vi "1000m_frame.vi"() -> ()   [LabVIEW 2017]
uses:
  <vilib>/gmath/NI_Gmath.lvlib
panel:
  out "normált eredõ SNR":cluster{dbl[], dbl[]}(graph)
  out "normált X SNR (+1 felharmonikus)":cluster{dbl[], dbl[]}(graph)
  out "normált X SNR":cluster{dbl[], dbl[]}(graph)
  out "r 8":dbl format="%.7g"
  out "r 7":dbl format="%.7g"
  out "r 6":dbl format="%.7g"
  out "r 5":dbl format="%.7g"
  out "r 4":dbl format="%.7g"
  out "r 3":dbl format="%.7g"
  out "r 2":dbl format="%.7g"
  out "r":dbl format="%.7g"
  out "impulse szum/mean":cluster{"X":dbl, "Y":dbl}[](graph)
  in  "felharmonikus N":i32=2
  in  "SNR window width [Hz]":dbl=0.2 format="%#_13g"
  out "impulse mean":cluster{"X":dbl, "Y":dbl}[](graph)
  out "impulse szum":cluster{"X":dbl, "Y":dbl}[](graph)
  out "impulse sd":cluster{"X":dbl, "Y":dbl}[](graph)
  out "impulse szum/time (egész jó)":cluster{"X":dbl, "Y":dbl}[](graph)
  out "X SNR (+1 felharmonikus)":cluster{"X":dbl, "Y":dbl}[](graph)
  out "resultant SNR":cluster{"X":dbl, "Y":dbl}[](graph)
  out "X SNR":cluster{"X":dbl, "Y":dbl}[](graph)
  in  "Path":path=path "C:/Users/Lenovo/Desktop/szakdoga/data/pálya/1000m"
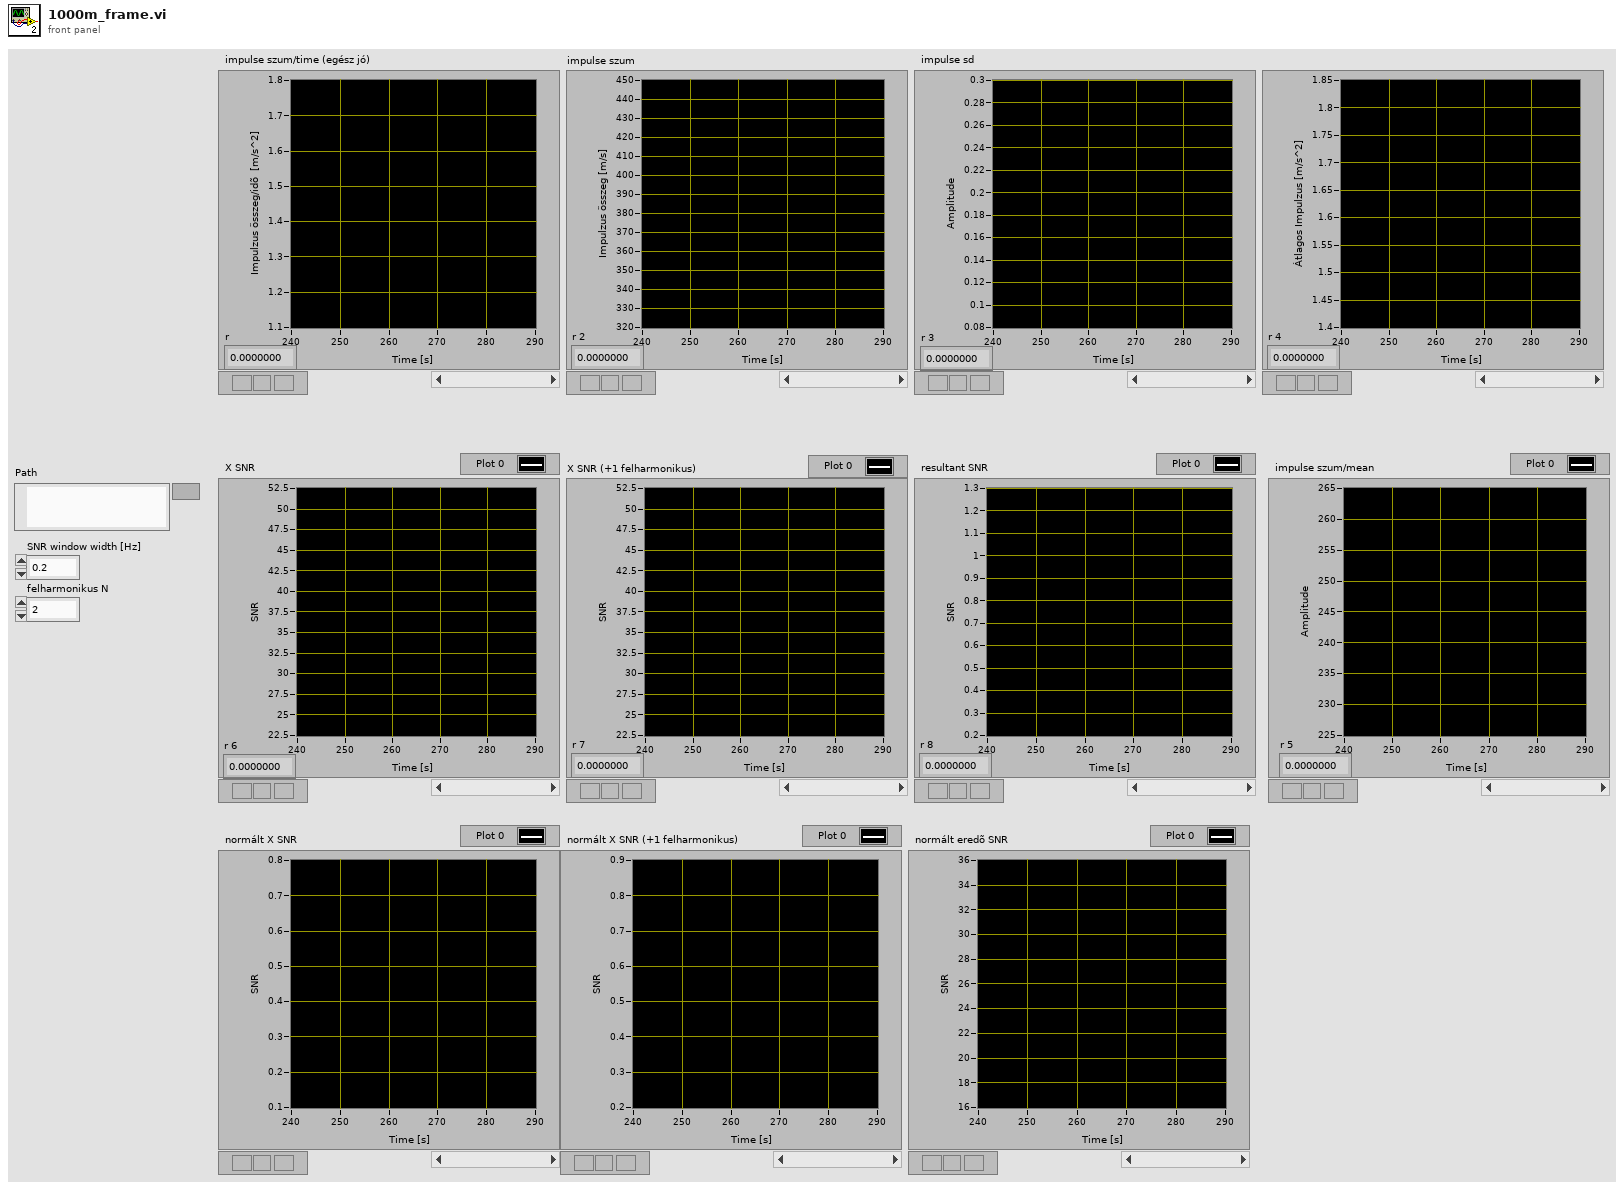
[diagram p1: front panel]
types:
  T1 = cluster{cluster{dbl, "impulse szum/time":dbl}[], cluster{dbl, "impulse  szum":dbl}[], cluster{dbl, "impulse standard deviation":dbl}[], cluster{dbl, "impulse mean":dbl}[], cluster{dbl, "X SNR 1":dbl}[], cluster{dbl, "X SNR 2":dbl}[], cluster{dbl, "X SNR 3":dbl}[], cluster{dbl, "impulse szum/avg":dbl}[]}
  T2 = cluster{cluster{dbl, dbl}[], cluster{dbl, "impulse  szum":dbl}[], cluster{dbl, "impulse standard deviation":dbl}[], cluster{dbl, "impulse mean":dbl}[], cluster{dbl, dbl}[], cluster{dbl, dbl}[], cluster{dbl, dbl}[], cluster{dbl, "impulse szum/mean":dbl}[]}
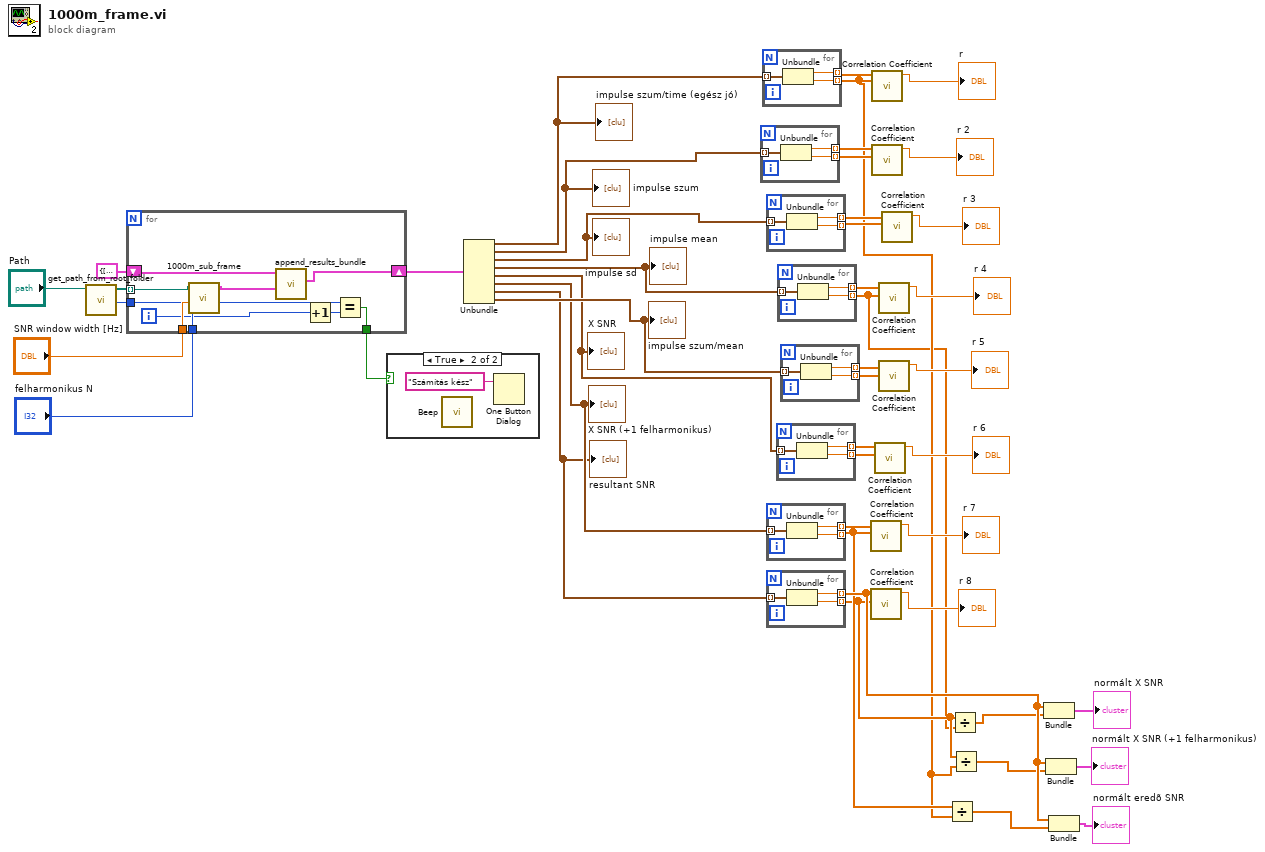
[diagram p0: block diagram]
diagram:
  n1 = call "get_path_from_root_folder.vi"("Path"="Path") -> ("Number of Files"=w42:i32, "Array"=w46:path[])  [unwired: 9 in]
  n2 = for {
    tunnel: w46 -> [w54] mode=indexing
    tunnel: "SNR window width [Hz]" -> [w52]
    tunnel: "felharmonikus N" -> [w51]
    tunnel: w42 -> [w50]
    tunnel: [w47] -> w41
    shift-right: [w55] -> w39
    shift-left: T1 {[], [], [], [], [], [], [], []} ("concat(X,Y)") -> [w56]
    i -> [w48]
    n3 = call "1000m_sub_frame.vi"("felharmonikus N"=w51, "SNR window width [Hz]"=w52, "path to binary file"=w54) -> ("output cluster"=w53:T2)  [unwired: 8 in]
    n4 = call "append_results_bundle.vi"("Y"=w53, "X"=w56) -> ("concat(X,Y)"=w55:T1)  [unwired: 8 in]
    n5 = Increment(x=w48) -> (x+1=w49:i32)
    n6 = Equal?(x=w50, y=w49) -> (x = y?=w47:bool)
  }
  n7 = case shown="True" w41 {
    frame False {
    }
    frame True {
      n8 = call <vilib>:"Beep.vi"() -> ()  [unwired: 12 in]
      n9 = One Button Dialog(message="Számítás kész") -> ()  [unwired: 1 in, 1 out]
    }
  }
  n10 = Unbundle(w39) -> (w38:cluster{dbl, "impulse szum/time":dbl}[], w37:cluster{dbl, "impulse  szum":dbl}[], w36:cluster{dbl, "impulse standard deviation":dbl}[], w35:cluster{dbl, "impulse mean":dbl}[], w33:cluster{dbl, "X SNR 1":dbl}[], w32:cluster{dbl, "X SNR 2":dbl}[], w31:cluster{dbl, "X SNR 3":dbl}[], w34:cluster{dbl, "impulse szum/avg":dbl}[])
  "X SNR" <- w33
  "resultant SNR" <- w31
  "X SNR (+1 felharmonikus)" <- w32
  "impulse szum/time (egész jó)" <- w38
  "impulse sd" <- w36
  "impulse szum" <- w37
  "impulse mean" <- w35
  "impulse szum/mean" <- w34
  n11 = for {
    tunnel: w37 -> [w60] mode=indexing
    tunnel: [w59] -> w26 mode=indexing
    tunnel: [w58] -> w4 mode=indexing
    n12 = Unbundle(w60) -> (w59:dbl, "impulse  szum"=w58:dbl)
  }
  n13 = for {
    tunnel: w38 -> [w63] mode=indexing
    tunnel: [w62] -> w30 mode=indexing
    tunnel: [w61] -> w2 mode=indexing
    n14 = Unbundle(w63) -> (w62:dbl, "impulse szum/time"=w61:dbl)
  }
  n15 = for {
    tunnel: w36 -> [w66] mode=indexing
    tunnel: [w65] -> w18 mode=indexing
    tunnel: [w64] -> w5 mode=indexing
    n16 = Unbundle(w66) -> (w65:dbl, "impulse standard deviation"=w64:dbl)
  }
  n17 = for {
    tunnel: w32 -> [w69] mode=indexing
    tunnel: [w68] -> w15 mode=indexing
    tunnel: [w67] -> w7 mode=indexing
    n18 = Unbundle(w69) -> (w68:dbl, "X SNR 2"=w67:dbl)
  }
  n19 = for {
    tunnel: w31 -> [w72] mode=indexing
    tunnel: [w71] -> w11 mode=indexing
    tunnel: [w70] -> w6 mode=indexing
    n20 = Unbundle(w72) -> (w71:dbl, "X SNR 3"=w70:dbl)
  }
  n21 = for {
    tunnel: w33 -> [w75] mode=indexing
    tunnel: [w74] -> w17 mode=indexing
    tunnel: [w73] -> w16 mode=indexing
    n22 = Unbundle(w75) -> (w74:dbl, "X SNR 1"=w73:dbl)
  }
  n23 = for {
    tunnel: w35 -> [w78] mode=indexing
    tunnel: [w77] -> w28 mode=indexing
    tunnel: [w76] -> w1 mode=indexing
    n24 = Unbundle(w78) -> (w77:dbl, "impulse mean"=w76:dbl)
  }
  n25 = for {
    tunnel: w34 -> [w81] mode=indexing
    tunnel: [w80] -> w27 mode=indexing
    tunnel: [w79] -> w3 mode=indexing
    n26 = Unbundle(w81) -> (w80:dbl, "impulse szum/avg"=w79:dbl)
  }
  n27 = call <vilib>:"Correlation Coefficient.vi"("Y"=w7, "X"=w15) -> ("correlation coefficient r"=→"r 7":dbl)  [unwired: 8 in, 1 out]
  n28 = call <vilib>:"Correlation Coefficient.vi"("Y"=w6, "X"=w11) -> ("correlation coefficient r"=→"r 8":dbl)  [unwired: 8 in, 1 out]
  n29 = call <vilib>:"Correlation Coefficient.vi"("Y"=w2, "X"=w30) -> ("correlation coefficient r"=→"r":dbl)  [unwired: 8 in, 1 out]
  n30 = call <vilib>:"Correlation Coefficient.vi"("Y"=w4, "X"=w26) -> ("correlation coefficient r"=→"r 2":dbl)  [unwired: 8 in, 1 out]
  n31 = call <vilib>:"Correlation Coefficient.vi"("Y"=w16, "X"=w17) -> ("correlation coefficient r"=→"r 6":dbl)  [unwired: 8 in, 1 out]
  n32 = call <vilib>:"Correlation Coefficient.vi"("Y"=w1, "X"=w28) -> ("correlation coefficient r"=→"r 4":dbl)  [unwired: 8 in, 1 out]
  n33 = call <vilib>:"Correlation Coefficient.vi"("Y"=w3, "X"=w27) -> ("correlation coefficient r"=→"r 5":dbl)  [unwired: 8 in, 1 out]
  n34 = call <vilib>:"Correlation Coefficient.vi"("Y"=w5, "X"=w18) -> ("correlation coefficient r"=→"r 3":dbl)  [unwired: 8 in, 1 out]
  n35 = Divide(x=w7, y=w2) -> (x/y=w8:dbl[])
  n36 = Divide(x=w6, y=w1) -> (x/y=w10:dbl[])
  n37 = Divide(x=w6, y=w2) -> (x/y=w9:dbl[])
  n38 = Bundle(w11, w10) -> (→"normált X SNR":cluster{dbl[], dbl[]})  [unwired: 1 in]
  n39 = Bundle(w11, w9) -> (→"normált X SNR (+1 felharmonikus)":cluster{dbl[], dbl[]})  [unwired: 1 in]
  n40 = Bundle(w11, w8) -> (→"normált eredõ SNR":cluster{dbl[], dbl[]})  [unwired: 1 in]
